vi "Copy Client Library.vi"(8 "error in":errorcluster, 10 "client name":string, 11 "project ref":refnum<vi>) -> (0 "error out":errorcluster, 2 "measure vi refnum":refnum<vi>, 3 "project ref out":refnum<vi>)   [LabVIEW 2021, in "MeasurementClient Editor.lvlib"]
uses:
  MeasurementClient Editor.lvlib
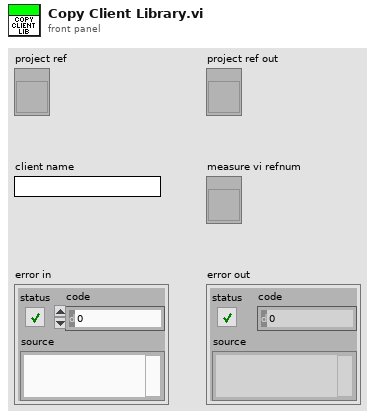
[diagram p1: front panel]
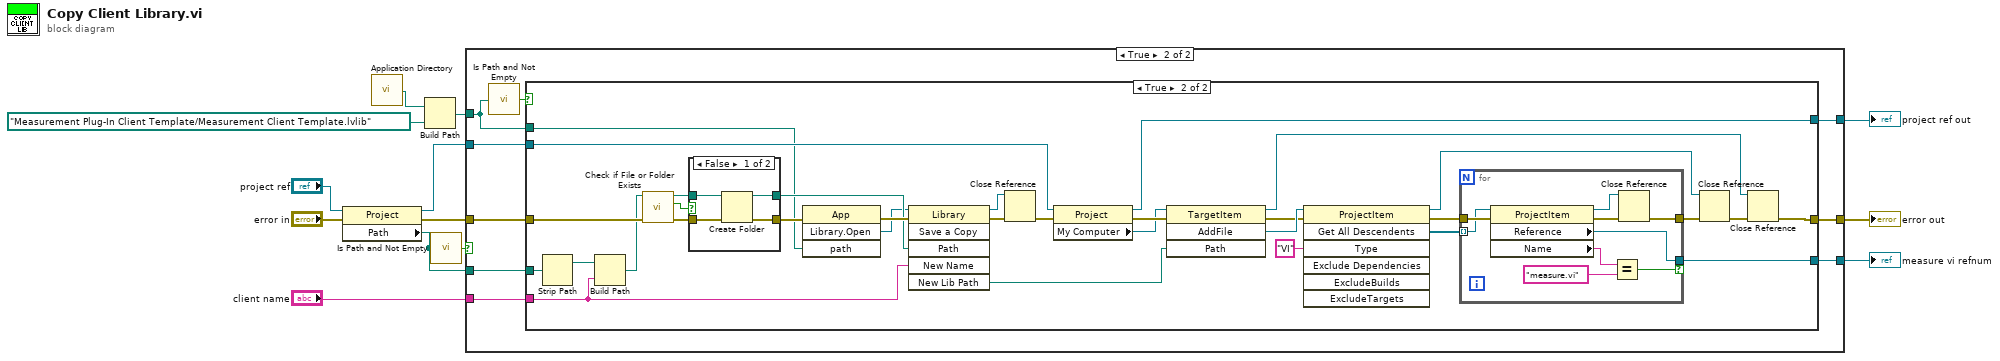
[diagram p0: block diagram]
diagram:
  n1 = property class="Project"(reference="project ref", error in="error in") -> (reference out=w4:refnum<vi>, error out=w12:errorcluster, "Path"=w8:path)
  n2 = call <vilib>:"Application Directory.vi"() -> ("Application Directory"=w9:path)
  n3 = Build Path(base path=w9, name or relative path=path "Measurement Plug-In Client Template/Measurement Client Template.lvlib") -> (appended path=w6:path)
  n4 = call <vilib>:"Is Path and Not Empty.vi"("path"=w8) -> ("Is Path and Not Empty?"=w10:bool)  [unwired: 4 in]
  n5 = case shown="True" w10 {
    tunnel: w12 -> [w15 w24]
    tunnel: w6 -> [_ w17]
    tunnel: w8 -> [_ w23]
    tunnel: "client name" -> [_ w22]
    tunnel: w4 -> [w14 w21]
    tunnel: [w15 w20] -> w3
    tunnel: [w14 w19] -> w2
    tunnel: [_ w18] -> w1
    frame False {
    }
    frame True {
      n6 = call <vilib>:"Is Path and Not Empty.vi"("path"=w17) -> ("Is Path and Not Empty?"=w16:bool)  [unwired: 4 in]
      n7 = case shown="True" w16 {
        tunnel: w24 -> [w26 w58]
        tunnel: w23 -> [_ w56]
        tunnel: w22 -> [_ w48]
        tunnel: w21 -> [w25 w46]
        tunnel: [w26 w32] -> w20
        tunnel: [w25 w30] -> w19
        tunnel: [_ w28] -> w18
        tunnel: w17 -> [_ w27]
        frame False {
        }
        frame True {
          n8 = Strip Path(path=w56) -> (stripped path=w55:path)  [unwired: 1 out]
          n9 = Build Path(base path=w55, name or relative path=w48) -> (appended path=w54:path)
          n10 = call <vilib>:"Check if File or Folder Exists.vi"("error in (no error)"=w58, "path"=w54) -> ("error out"=w53:errorcluster, "file or folder exists?"=w52:bool, "dup path"=w51:path)  [unwired: 7 in]
          n11 = case shown="False" w52 {
            tunnel: w53 -> [w71 w72]
            tunnel: w51 -> [w70 w73]
            tunnel: [w69 w72] -> w49
            tunnel: [w68 w73] -> w50
            frame False {
              n12 = Create Folder(path (use dialog)=w70, error in=w71) -> (created path=w68:path, error out=w69:errorcluster)  [unwired: 1 in, 1 out]
            }
            frame True {
            }
          }
          n13 = invoke class="App" method="Library.Open"(error in=w49, "path"=w27) -> (error out=w57:errorcluster, "Open Library"=w47:refnum<vi>)  [unwired: 2 in, 2 out]
          n14 = invoke class="Library" method="Save a Copy"(reference=w47, error in=w57, "Path"=w50, "New Name"=w48) -> (reference out=w43:refnum<vi>, error out=w44:errorcluster, "New Lib Path"=w41:path)  [unwired: 2 in, 3 out]
          n15 = Close Reference(reference=w43, error in (no error)=w44) -> (error out=w45:errorcluster)
          n16 = property class="Project"(reference=w46, error in=w45) -> (reference out=w30:refnum<vi>, error out=w42:errorcluster, "My Computer"=w31:refnum<vi>)
          n17 = invoke class="TargetItem" method="AddFile"(reference=w31, error in=w42, "Path"=w41) -> (reference out=w34:refnum<vi>, error out=w39:errorcluster, "AddFile"=w40:refnum<vi>)  [unwired: 1 in, 1 out]
          n18 = invoke class="ProjectItem" method="Get All Descendents"(reference=w40, error in=w39, "Type"="VI") -> (reference out=w33:refnum<vi>, error out=w37:errorcluster, "All Descendents"=w36:refnum<vi>[])  [unwired: 4 in, 4 out]
          n19 = for {
            tunnel: w37 -> [w67]
            tunnel: w36 -> [w66] mode=indexing
            tunnel: [w63] -> w28 if=w62
            tunnel: [w60] -> w29
            n20 = property class="ProjectItem"(reference=w66, error in=w67) -> (reference out=w65:refnum<vi>, error out=w61:errorcluster, "Reference"=w63:refnum<vi>, "Name"=w64:string)
            n21 = Equal?(x=w64, y="measure.vi") -> (x = y?=w62:bool)
            n22 = Close Reference(reference=w65, error in (no error)=w61) -> (error out=w60:errorcluster)
          }
          n23 = Close Reference(reference=w33, error in (no error)=w29) -> (error out=w35:errorcluster)
          n24 = Close Reference(reference=w34, error in (no error)=w35) -> (error out=w32:errorcluster)
        }
      }
    }
  }
  "error out" <- w3
  "project ref out" <- w2
  "measure vi refnum" <- w1
